vi "3458A Check Needed Aux HW.vi"(3 "digitizer session":T1 {"channels"."Range [Vpk]" min=0.0}) -> (14 "uses AWG clocking?":bool, 15 "SLAVEs clocked by AWG?":bool, 16 "SLAVEs clocked from TIMER?":bool, 17 "uses counter?":bool, 18 "uses counter for delta T sync?":bool, 19 "uses counter for DFLL?":bool)   [LabVIEW 2013, in "3458A Virtual Digitizer.lvlib"]
doc: "Checks measurement session and returnes various flags specifying which auxiliary instruments are used for selected mode of synchonization (AWG, Counter)."
uses:
  3458A Virtual Digitizer.lvlib
  3458A Digitizer Session.ctl
  3458A Virtual Channel Config.ctl
  Counter/Counter Session.ctl
  Counter/Counter Type.ctl
  AWG/AWG Session.ctl
  AWG/AWG Type.ctl
  3458A Sync Mode.ctl
  3458A Idn Mode.ctl
  3458A Digitizing Low Levels/Configure/Sampling Mode.ctl
  3458A Digitizing Process Options.ctl
  3458A Data Packet.ctl
  3458A Aux Record Data.ctl
  3458A Digitizing Low Levels/Configure/Level Setup.ctl
  3458A Digitizing Low Levels/Configure/First Sample Trigger.ctl
  3458A Aperture Selection Mode.ctl
  Counter/Counter.lvlib
  AWG/AWG.lvlib
  3458A Digitizing Low Levels/3458A Digitizing Low Levels.lvlib
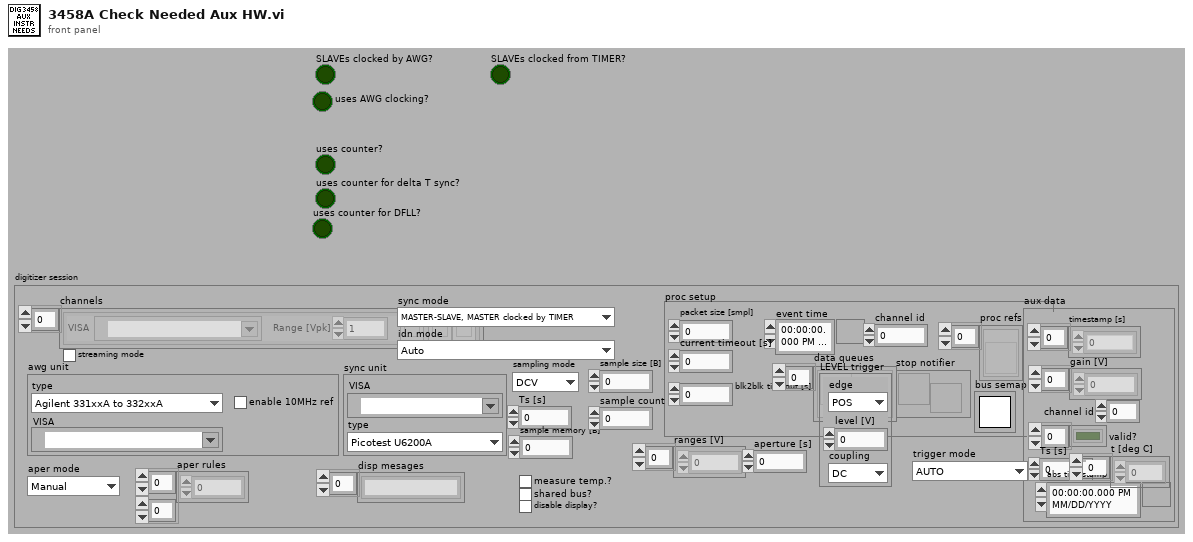
[diagram p1: front panel]
types:
  T1 = typedef "3458A Virtual Digitizer.lvlib/3458A Digitizer Session.ctl" = cluster{"channels":T2[], "sync unit":T3, "awg unit":T5, "sync mode":T7, "streaming mode":bool, "idn mode":T8, "sampling mode":T9, "Ts [s]":dbl, "sample memory [B]":i32, "proc setup":T10, "sample size [B]":i32, "sample count":i32, "aux data":T12, "ranges [V]":dbl[], "aperture [s]":dbl, "LEVEL trigger":T13, "trigger mode":T14, "measure temp.?":bool, "disp mesages":string[], "shared bus?":bool, "disable display?":bool, "aper mode":T15, "aper rules":dbl[][]}
  T2 = typedef "3458A Virtual Digitizer.lvlib/3458A Virtual Channel Config.ctl" = cluster{"VISA":refnum<visa-resource-name>, "Range [Vpk]":dbl, "btn clr":bool, "btn up":bool, "btn down":bool}
  T3 = typedef "Counter.lvlib/Counter Session.ctl" = cluster{"VISA":refnum<visa-resource-name>, "type":T4}
  T4 = typedef "Counter.lvlib/Counter Type.ctl" = enum16{"Picotest U6200A", "dummy"}
  T5 = typedef "AWG.lvlib/AWG Session.ctl" = cluster{"type":T6, "VISA":refnum<visa-resource-name>, "enable 10MHz ref":bool}
  T6 = typedef "AWG.lvlib/AWG Type.ctl" = enum16{"Agilent 331xxA to 332xxA", "Agilent 335xxA to 336xxA", "Tektronix AFG3101C", "dummy"}
  T7 = typedef "3458A Virtual Digitizer.lvlib/3458A Sync Mode.ctl" = enum16{"MASTER-SLAVE, MASTER clocked by TIMER", "MASTER-SLAVE, MASTER clocked by AWG", "ALL clocked by AWG", "MASTER-SLAVE, ALL clocked by TIMER", "ALL clocked by AWG with DFLL"}
  T8 = typedef "3458A Virtual Digitizer.lvlib/3458A Idn Mode.ctl" = enum16{"Auto", "Sequential (chn A, chn B, ...)", "From calibration string"}
  T9 = typedef "3458A Virtual Digitizer.lvlib/3458A Digitizing Low Levels.lvlib/Sampling Mode.ctl" = enum16{"DCV", "DSDC", "DSAC"}
  T10 = typedef "3458A Virtual Digitizer.lvlib/3458A Digitizing Process Options.ctl" = cluster{"channel id":i32, "packet size [smpl]":i32, "current timeout [s]":dbl, "blk2blk timeout [s]":dbl, "event time":timestamp, "stop notifier":refnum<notifier>, "data queues":refnum<queue>[], "proc refs":refnum<vi>[], "bus semaphore":T11}
  T11 = typedef "Semaphore RefNum" = refnum<k1>
  T12 = typedef "3458A Virtual Digitizer.lvlib/3458A Aux Record Data.ctl" = cluster{"channel id":i32, "valid?":bool[], "gain [V]":dbl[], "timestamp [s]":dbl[], "Ts [s]":dbl, "abs timestamp":timestamp, "t [deg C]":dbl[]}
  T13 = typedef "3458A Virtual Digitizer.lvlib/3458A Digitizing Low Levels.lvlib/Level Setup.ctl" = cluster{"edge":enum16{"POS", "NEG"}, "level [V]":dbl, "coupling":enum16{"DC", "AC"}}
  T14 = typedef "3458A Virtual Digitizer.lvlib/3458A Digitizing Low Levels.lvlib/First Sample Trigger.ctl" = enum16{"AUTO", "EXT", "SYN", "SGL", "HOLD", "LEVEL"}
  T15 = typedef "3458A Virtual Digitizer.lvlib/3458A Aperture Selection Mode.ctl" = enum16{"Manual", "Maximum", "Table"}
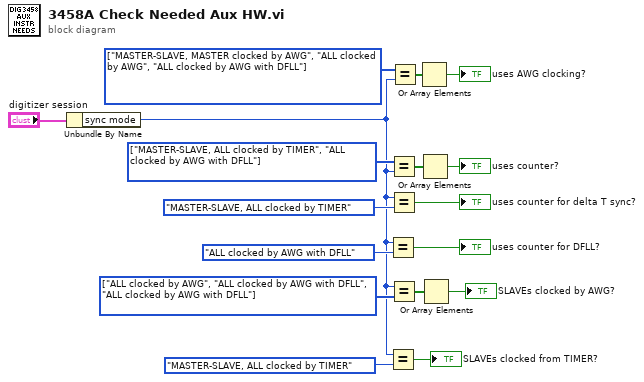
[diagram p0: block diagram]
diagram:
  w6 = T7[] [enum."ALL clocked by AWG", enum."ALL clocked by AWG with DFLL", enum."ALL clocked by AWG with DFLL"] items=["MASTER-SLAVE, MASTER clocked by TIMER", "MASTER-SLAVE, MASTER clocked by AWG", "ALL clocked by AWG", "MASTER-SLAVE, ALL clocked by TIMER", "ALL clocked by AWG with DFLL"]
  w12 = T7[] [enum."MASTER-SLAVE, ALL clocked by TIMER", enum."ALL clocked by AWG with DFLL"] items=["MASTER-SLAVE, MASTER clocked by TIMER", "MASTER-SLAVE, MASTER clocked by AWG", "ALL clocked by AWG", "MASTER-SLAVE, ALL clocked by TIMER", "ALL clocked by AWG with DFLL"]
  w15 = T7[] [enum."MASTER-SLAVE, MASTER clocked by AWG", enum."ALL clocked by AWG", enum."ALL clocked by AWG with DFLL"] items=["MASTER-SLAVE, MASTER clocked by TIMER", "MASTER-SLAVE, MASTER clocked by AWG", "ALL clocked by AWG", "MASTER-SLAVE, ALL clocked by TIMER", "ALL clocked by AWG with DFLL"]
  n1 = Unbundle By Name("digitizer session") -> ("sync mode"=w3:T7)
  n2 = Equal?(x=w3, y=3458A_Sync_Mode."ALL clocked by AWG with DFLL") -> (x = y?=→"uses counter for DFLL?":bool)
  n3 = Equal?(x=w3, y=3458A_Sync_Mode."MASTER-SLAVE, ALL clocked by TIMER") -> (x = y?=→"SLAVEs clocked from TIMER?":bool)
  n4 = Equal?(x=w12, y=w3) -> (x = y?=w13:bool[])
  n5 = Equal?(x=w3, y=3458A_Sync_Mode."MASTER-SLAVE, ALL clocked by TIMER") -> (x = y?=→"uses counter for delta T sync?":bool)
  n6 = Equal?(x=w3, y=w6) -> (x = y?=w5:bool[])
  n7 = Equal?(x=w15, y=w3) -> (x = y?=w16:bool[])
  n8 = Or Array Elements(Boolean array=w16) -> (logical OR=→"uses AWG clocking?":bool)
  n9 = Or Array Elements(Boolean array=w13) -> (logical OR=→"uses counter?":bool)
  n10 = Or Array Elements(Boolean array=w5) -> (logical OR=→"SLAVEs clocked by AWG?":bool)
